vi "FindCenter.vi"(11 "Array in":i32[][](array[numeric])) -> (3 "Center":dbl[](array[numeric]))   [LabVIEW 2017]
uses:
  <vilib>/Analysis/Matrix/Numeric/Conversions/Array To Matrix - RA.vi
  <vilib>/Analysis/Matrix/Numeric/Conversions/Array To Matrix - RA2.vi
  <vilib>/Analysis/7linalg.llb/Solve Linear Equations (multiple right hand).vi
  <vilib>/Analysis/Matrix/Numeric/Conversions/Matrix To Array - RM.vi
  <vilib>/Analysis/Matrix/NI_Matrix.lvlib
  <vilib>/Analysis/NI_AALPro.lvlib
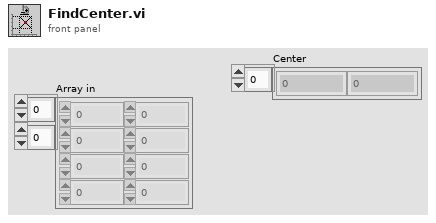
[diagram p1: front panel]
types:
  T1 = typedef "NI_Matrix.lvlib/RealMatrix.ctl" = dbl[][]
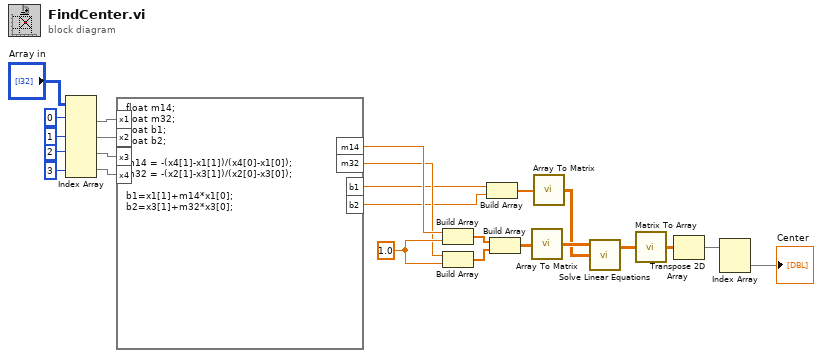
[diagram p0: block diagram]
diagram:
  w15 = 1.0
  n1 = Index Array(array="Array in", index (row) #1=0 ("index (row)"), index (row) #2=1 ("index (row)"), index (row) #3=2 ("index (row)"), index (row) #4=3 ("index (row)")) -> (element #1=w21:i32[], element #2=w22:i32[], element #3=w23:i32[], element #4=w24:i32[])  [unwired: 4 in]
  n2 = formula code="float m14;\nfloat m32;\nfloat b1;\nfloat b2;\n\nm14 = -(x4[1]-x1[1])/(x4[0]-x1[0]);\nm32 = -(x2[1]-x3[1])/(x2[0]-x3[0]);\n\nb1=x1[1]+m14*x1[0];\nb2=x3[1]+m32*x3[0];"("x1"=w21, "x2"=w22, "x3"=w23, "x4"=w24) -> ("m14"=w14:dbl, "m32"=w13:dbl, "b1"=w9:dbl, "b2"=w8:dbl)
  n3 = Build Array(w14, w15) -> (w12:dbl[])
  n4 = Build Array(w13, w15) -> (w11:dbl[])
  n5 = Build Array(w9, w8) -> (w7:dbl[])
  n6 = Build Array(w12, w11) -> (w10:dbl[][])
  n7 = call-poly <vilib>:"Array To Matrix.vi"("Real 2D Array"=w10) -> ("Real Matrix"=w6:T1)
  n8 = call-poly <vilib>:"Array To Matrix.vi"("Real 1D Array"=w7) -> ("Real Matrix (Column Vector)"=w5:T1)
  n9 = call-poly <vilib>:"Solve Linear Equations.vi"("Known Matrix"=w5, "Input Matrix"=w6) -> ("Solution Matrix"=w4:T1)  [unwired: 1 in, 1 out]
  n10 = call-poly <vilib>:"Matrix To Array.vi"("Real Matrix"=w4) -> ("Real 2D Array"=w3:dbl[][])
  n11 = Transpose 2D Array(2D array=w3) -> (transposed array=w2:dbl[][])
  n12 = Index Array(array=w2) -> (element=→"Center":dbl[])  [unwired: 2 in]
